vi "APG.vi"(0 "System no.":i32=1 min=1 max=4 step=1, 2 "NexlineChannels":string[](array[string]), 3 "All channels?":bool, 4 "Channel identifier?":bool=TRUE, 5 "error in":errorcluster) -> (19 "error out":errorcluster)   [LabVIEW 2020]
doc: "Auto Piezo Gain calibration of specified Nexline channels.\n\nE-755: If All channels = TRUE, then Channel identifier must be FALSE. Command not available for E-755.101. Use #7.vi to check if calibration has finished. To save the calibration parameters to default use \"PGS.vi\". See E-755 user manual for details."
panel:
  # "Auto Piezo Gain calibration of specified Nexline\nchannels."
  # "If all channels: use"
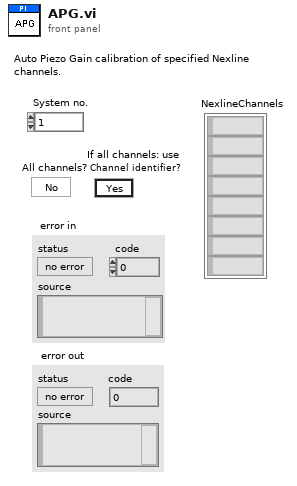
[diagram p1: front panel]
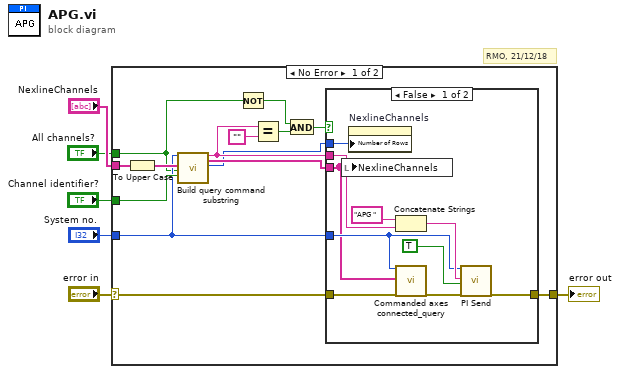
[diagram p0: block diagram]
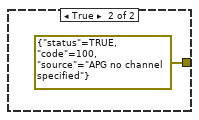
[diagram p2: hidden frame]
diagram:
  # "RMO, 21/12/18"
  n1 = case shown="No Error" "error in" {
    selector: "error in" -> [w9 w32]
    tunnel: "NexlineChannels" -> [w20 _]
    tunnel: "Channel identifier?" -> [w17 _]
    tunnel: "System no." -> [w15 _]
    tunnel: "All channels?" -> [w11 _]
    tunnel: [w8 w32] -> w2
    frame No Error {
      n2 = To Upper Case(1:w20) -> (0:w18:string[])
      n3 = call "Build query command substring.vi"("System no."=w15, "Axes to query in"=w18, "Query\nAll axes?"=w11, "For all axes: use\nAxis identifier?"=w17) -> ("Command substring"=w16:string, "Axes to query out"=w14:string[], "Number of rows"=w13:u32)  [unwired: 2 in, 11 out]
      n4 = Not(x=w11) -> (.not. x?=w10:bool)
      n5 = Equal?(x=w16, y="" ("x")) -> (x = y?=w12:bool)
      n6 = And(x=w10, y=w12) -> (x .and. y?=w7:bool)
      n7 = case shown="False" w7 {
        tunnel: w16 -> [w27 _]
        tunnel: w15 -> [w26 _]
        tunnel: w14 -> [w25 _]
        tunnel: w13 -> [w23 _]
        tunnel: w9 -> [w22 _]
        tunnel: [w21 errorcluster {"status"=TRUE, "code"=100, "source"="APG no channel specified"} ("error out")] -> w8
        frame False {
          n8 = local write "NexlineChannels"(w25) -> ()
          n9 = property on="NexlineChannels" class="Arr (strict)"("Number of Rows"=w23) -> ()  [unwired: 2 in, 2 out]
          n10 = Concatenate Strings("APG ", w27) -> (w28:string)
          n11 = call "Commanded axes connected_query.vi"("System no."=w26, "Commanded axes"=w25, "error in"=w22) -> ("error out"=w24:errorcluster)  [unwired: 1 in, 15 out]
          n12 = call "PI Send.vi"("System no."=w26, "String to send"=w28, "Attach termination char.?"=TRUE ("Attach Linefeed?"), "error in"=w24) -> ("error out"=w21:errorcluster)  [unwired: 2 in, 13 out]
        }
        frame True {
        }
      }
    }
    frame Error {
    }
  }
  "error out" <- w2
